vi "LC1_Global.vi"() -> ()   [LabVIEW 2016]
panel:
  out "LC1_WatchDogTimer Enable":bool
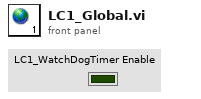
[diagram p1: front panel]
diagram:
